vi "Default Theme Info Entry Value-String.vi"(11 "Theme Info Entry":T1) -> (3 "Theme Info Entry Default Value":string)   [LabVIEW 2021, in "Appearance Actor.lvlib" / "Generic Theme.lvclass"]
doc: "For a given <B>Theme Info Entry</B>, returns the corresponding default value (String)."
uses:
  Generic Theme.lvclass
  Typedefs/Theme Info Entry--enum.ctl
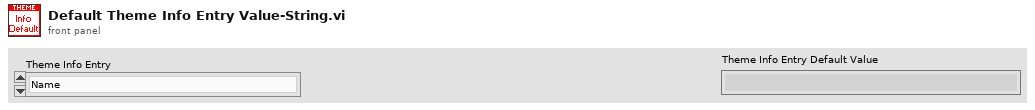
[diagram p1: front panel]
types:
  T1 = typedef "Appearance Actor.lvlib/Generic Theme.lvclass/Theme Info Entry--enum.ctl" = enum16{"Name", "Type", "Version"}
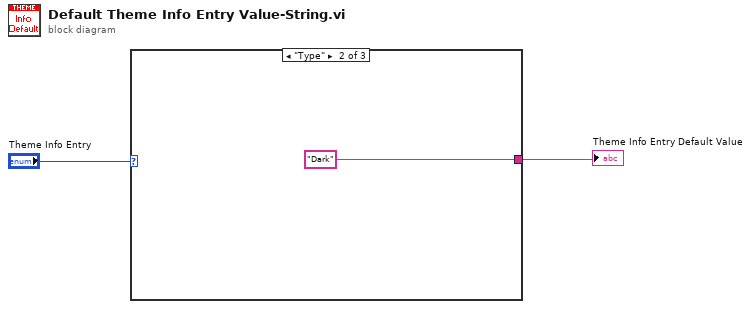
[diagram p0: block diagram]
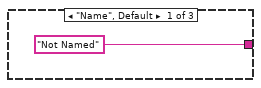
[diagram p2: hidden frame]
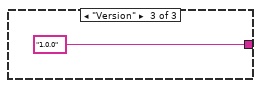
[diagram p3: hidden frame]
diagram:
  n1 = case shown="\"Type\"" "Theme Info Entry" {
    tunnel: ["Not Named" "Dark" "1.0.0"] -> w1
    frame "Name", Default {
    }
    frame "Type" {
    }
    frame "Version" {
    }
  }
  "Theme Info Entry Default Value" <- w1
